vi "RichToFlatrfcontrol_SetRFDCCalibrationCoefficientsResponse.vi"(5 "OutputClusterType":T1, 11 "InputCluster":T2) -> (3 "OutputCluster":T1)   [LabVIEW 2024, in "FlexSDR_gRPC_client.lvlib"]
uses:
  rfcontrol_SetRFDCCalibrationCoefficientsResponse.ctl
  rfcontrol_SetRFDCCalibrationCoefficientsResponse_Flat.ctl
  FlexSDR_gRPC_client.lvlib
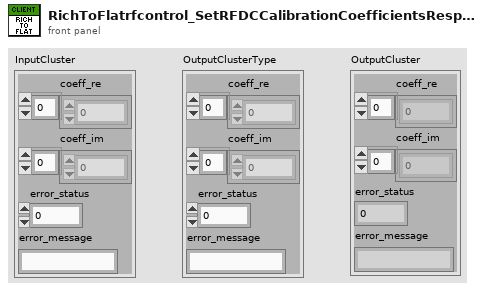
[diagram p1: front panel]
types:
  T1 = typedef "FlexSDR_gRPC_client.lvlib/rfcontrol_SetRFDCCalibrationCoefficientsResponse_Flat.ctl" = cluster{"coeff_re":i32[], "coeff_im":i32[], "error_status":i32, "error_message":string}
  T2 = typedef "FlexSDR_gRPC_client.lvlib/rfcontrol_SetRFDCCalibrationCoefficientsResponse.ctl" = cluster{"coeff_re":i32[], "coeff_im":i32[], "error_status":i32, "error_message":string}
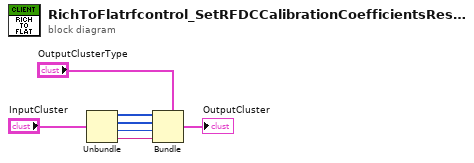
[diagram p0: block diagram]
diagram:
  n1 = Unbundle "Unbundle"("InputCluster") -> ("coeff_re"=w4:i32[], "coeff_im"=w3:i32[], "error_status"=w2:i32, "error_message"=w1:string)
  n2 = Bundle "Bundle"(cluster="OutputClusterType", "coeff_re"=w4, "coeff_im"=w3, "error_status"=w2, "error_message"=w1) -> (→"OutputCluster":T1)
